vi "Close Instrument Sessions.vi"(0 "Scalar Path Group in":refnum<class "Scalar Path Group.lvclass">, 11 "error in":errorcluster) -> (4 "Scalar Path Group out":refnum<class "Scalar Path Group.lvclass">, 15 "error out":errorcluster)   [LabVIEW 2023, in "RFFixtureCharact.Public.lvlib" / "Scalar Path Group.lvclass"]
uses:
  Scalar Path Group.lvclass
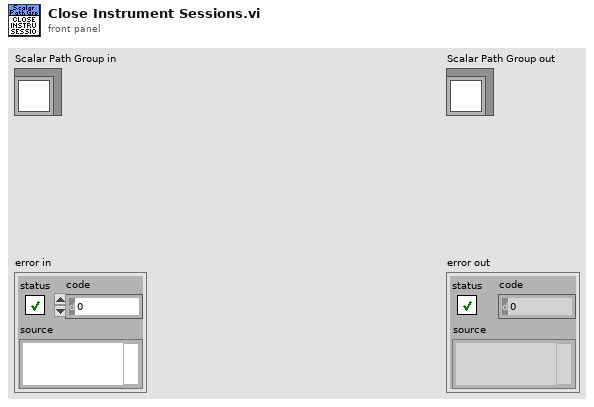
[diagram p1: front panel]
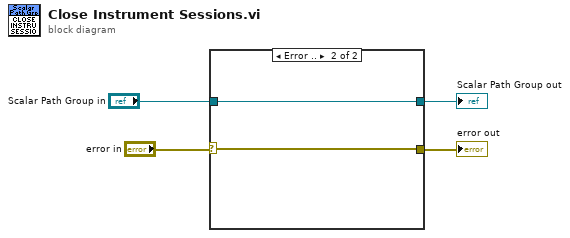
[diagram p0: block diagram]
diagram:
  n1 = case shown="Error .." "error in" {
    selector: "error in" -> [w6 w8]
    tunnel: [w6 w8] -> w3
    tunnel: [w5 w7] -> w2
    tunnel: "Scalar Path Group in" -> [w5 w7]
    frame No Error {
    }
    frame Error {
    }
  }
  "error out" <- w3
  "Scalar Path Group out" <- w2
